vi "CRYReplace Hardware Curve Name.vi"(6 "Hardware In":string, 8 "New Name":string, 9 "Old Name":string, 10 "Type In":enum16{"Add", "Delete", "Rename"}(ring), 11 "Is Input?":bool) -> ()   [LabVIEW 2013]
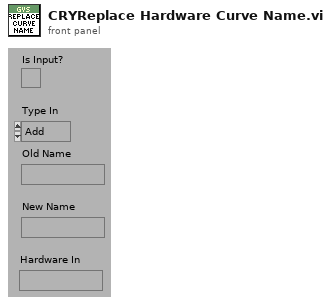
[diagram p1: front panel]
types:
  T1 = typedef "CRYStep.ctl" = cluster{"No.VI":i32, "Category":string, "StepName":string, "Seq setup flattened":string, "Comment":string, "Steps config.":bool[], "Jump config":i32[], "Start":dbl, "Increment":dbl, "Name":string, "Unit":string, "Y data":u16, "Y prefix":string, "Y dB ref":dbl, "Y unit":string, "Repeat State Array":cluster{"Start":dbl, "Increment":dbl, "Count":i32, "Num":i32}[]}
  T2 = typedef "CRYStimulus Cluster.ctl" = cluster{"StimulusType":string, "UseMLValArray":u16[], "ML_axisArray":u16[], "MLValLevelNameArray":string[], "Level(U)Array":dbl[], "Start(Stop)FreqArray":dbl[], "Start(Stop)AmpArray":dbl[], "StepResolutionArray":u16[], "Unit_Array":u16[], "DegValArray":dbl[], "DegUnitArray":string[], "Steps1":i32, "Cycle/step1(#)":u32, "Time/step1(s)":dbl, "Transition1":dbl, "SweepRate2":dbl, "Freq3(Hz)":dbl, "Steps3(#)":dbl, "Cycles3(#)":u32, "StepSize3":dbl, "wave time":string, "RMS_Value4":dbl, "Peak_Value4":dbl, "WavePath4":string, "RMS_unit4":string, "Peak_unit4":string, "wave Info":string, "dc_ctrl5_1":u16, "dc_ctrl5_2":u16, "dc_polar5":u16, "Max.Current":u16, "Steps5(#)":u32, "Time/Step5":dbl, "Level5":dbl, "StepsSize5Val":dbl, "StepSize5Unit":string, "SweepType":u16, "Fixed/Ratio6":u16, "Transition6":dbl, "Steps6(#)":dbl, "Cycle/Steps6(#)":u32, "Time/Steps6(s)":dbl, "Freq6(Hz)":dbl, "Difference6(Hz)":dbl, "Ratio6":string, "NoiseType7":u16, "Duration7(s)":dbl, "MinFreq7(Hz)":dbl, "MaxFreq7(Hz)":dbl, "MinFreq8(Hz)":dbl, "MaxFreq8(Hz)":dbl, "FreqRounding8":bool, "Duration8(s)":dbl, "Tones8":dbl, "RoundingVal8":dbl, "ApplyEQ":bool, "Duration(s)":dbl, "CustomStimulusName ":string, "Flatten Element Array":string[], "sine waves":cluster{"freq":dbl, "ampl":dbl, "cycles":dbl}[], "Channel Out":i32, "RatioVal6":dbl, "TabCtrl6":enum32{"Master Tone", "Slave Tone"}, "Signal Type Name":string, "Help":string, "Channel Sel":u16}
  T3 = typedef "CRYAcquisition Cluster.ctl" = cluster{"Mode":u16, "Name":string, "use ch name":bool, "Record Time":dbl, "hide rec":bool, "hide play":bool, "rec delay":dbl, "rec pad":dbl, "dcc units":i8, "sine gen setting":string, "scope_fft setting":string, "voltmeter setting":string, "rta setting":string, "trig offset(sec)":dbl, "triggered  record":bool, "trig level":dbl, "trig unit":u8, "trig slop":bool, "trig timeout(sec)":dbl, "add record":bool, "EQ":bool, "record table":string[][], "play table":string[][], "trig channel":string, "Help":string}
  T4 = typedef "CRYAnalysis Cluster.ctl" = cluster{"Name":string, "Harmonics":dbl[], " Algorithm":u16, "delay":dbl, "THD(%)":bool, "Rub&Buzz":bool, "Imp":bool, "Imp Ref resistor":dbl, "Y data":u16, "Y prefix":string, "Y unit":string, "Y dB ref":dbl, "Custom Curve Names":string[], "har list items":string[], "Envelope":bool, "use custom unit":bool, "autodelay ch":dbl, "impulse":bool, " start ms":dbl, " stop ms":dbl, "Scaling":i32, "Default Overlap ":bool, "Advanced View":bool, "Loose Particle":bool, "Use default":bool, "Auto-Correlation(Stimulus)":bool, "Auto-Correlation(Response)":bool, "Deconvolved Response":bool, "Mic Current":bool, "M List Vaiues":u16, "Type":u16, "Delay Method":u16, "Apply Correction Out":bool, "Apply Correction In":bool, "Harmonics @ meas.frq":bool, "THD Normalized(%)":bool, "Total Distortion":bool, "THD+Noise(%)":bool, "Rub&Buzz Norm'd(%)":bool, "Standard Error":bool, "Confidence Limits":bool, "Total Diff":bool, "Total Noise":bool, "Total DFD(%)":bool, "Total IMD(%)":bool, "Total IM":bool, "Total DFD+Noise(%)":bool, "Use Channel Name":bool, "Waveform In":string, "Waveform Out":string, "Method":u16, "Spectral Scaling":u16, "Appliied Unit":u16, "Length Unit":u16, "Applied Units":u16, "Sens Item":u16, "Tab":i32, "Distance Unit":u16, "discard cycles":dbl, "Weigting":string, "Averaging Time":dbl, "Max duration":dbl, "Min duration":dbl, "Attack Threshold":dbl, "Hysteresis Up":dbl, "Fmin(Hz)":dbl, "Fmax(Hz)":dbl, "Freq.Resolution":dbl, "Over-samples Res.":dbl, "Win Resolution":dbl, "distance":dbl, "samples":dbl, "Overlap":dbl, "Record Length":dbl, "No.of FFTs":dbl, "Hz":dbl, "record delay":dbl, " Std Err":dbl, "Response":bool, "Coherent Power*":bool, "Stimulus":bool, "Measurement Confidence":bool, "Auto Spectrum(Response)*":bool, "Auto Spectrum(Stimulus)*":bool, "Cross Spectrum*":bool, "functions":bool, "Frequency Response":bool, "Non-Coherent Power*":bool, "Coherence (%)":bool, "Non-Coherence (%)":bool, "Signal-Noise Ratio (dB)":bool, "Non-Coherenct Distirtion*":bool, "Result Waveforms":bool, "Coupling":bool, "Averaging":u16, "Harmonics":i32, "Custom Curve Names":i32, "unLabel":string, "Custom Curve Names":string, "Unit":string, "Total IMD + Noise(%) ":bool, "ResponseMe":u16, "Intermod":dbl[], "Diff\n":dbl[], "Cross-Correlation":bool, "IM list items":string[], "Diff list items":string[], "TSR Window Type":string, "Help":string, "Custom Curve IDs":i32[], "Default Curve Names":string[], "Loose Particle waveform":bool, "Perceptual Rub&Buzz":bool, "Imp Auto Mode":u16, "Mic Auto Mode":u16, "Mic Ref resistor":dbl, "Curve Resolution":u16, "Curve Resolution Hz":dbl, "Polarity":bool}
  T5 = typedef "CRYWaveform Cluster.ctl" = cluster{"Waveform":cluster{"X0":dbl, "dX":dbl, "Y":sgl[]}, "X data":u16, "Y data":u16, "Y axis":u16, "X unit":string, "Y unit":string, "Y dB ref":dbl, "display Y":bool, "display X":bool, "Overload?":bool, "Test Info":string, "Step No.":i32, "Name":string, "protected":bool, "Sqc history":string[], "Signal Channel ID":i32, "Plot Settings":cluster{"Color":u32, "Interpolation":u8, "Point Style":u8, "Line Style":u8, "Point Color":u32, "Line Width":u8, "Bar Plot Style":u8, "Fill To":i16}, "AutoProtect":bool}
  T6 = typedef "CRYStimulus Test Infor Cluster.ctl" = cluster{"Stimulus Type":string, "Signal Type":string, "In/Out":bool, "FAPS":cluster{"freq":dbl, "ampl":dbl, "cycles":dbl, "samples":i32}[], "Sampling Rate":dbl, "Samples":i32, "Analysis Param":string, "Resolution":u16, "Steps":u32, "Analysis Value":dbl[], "Diff Freq":dbl, "FStart":dbl, "FStop":dbl, "Calibration Param":string, "Anti Alias":dbl, "Level Out1":dbl, "Level Out2":dbl, "EQ":bool}
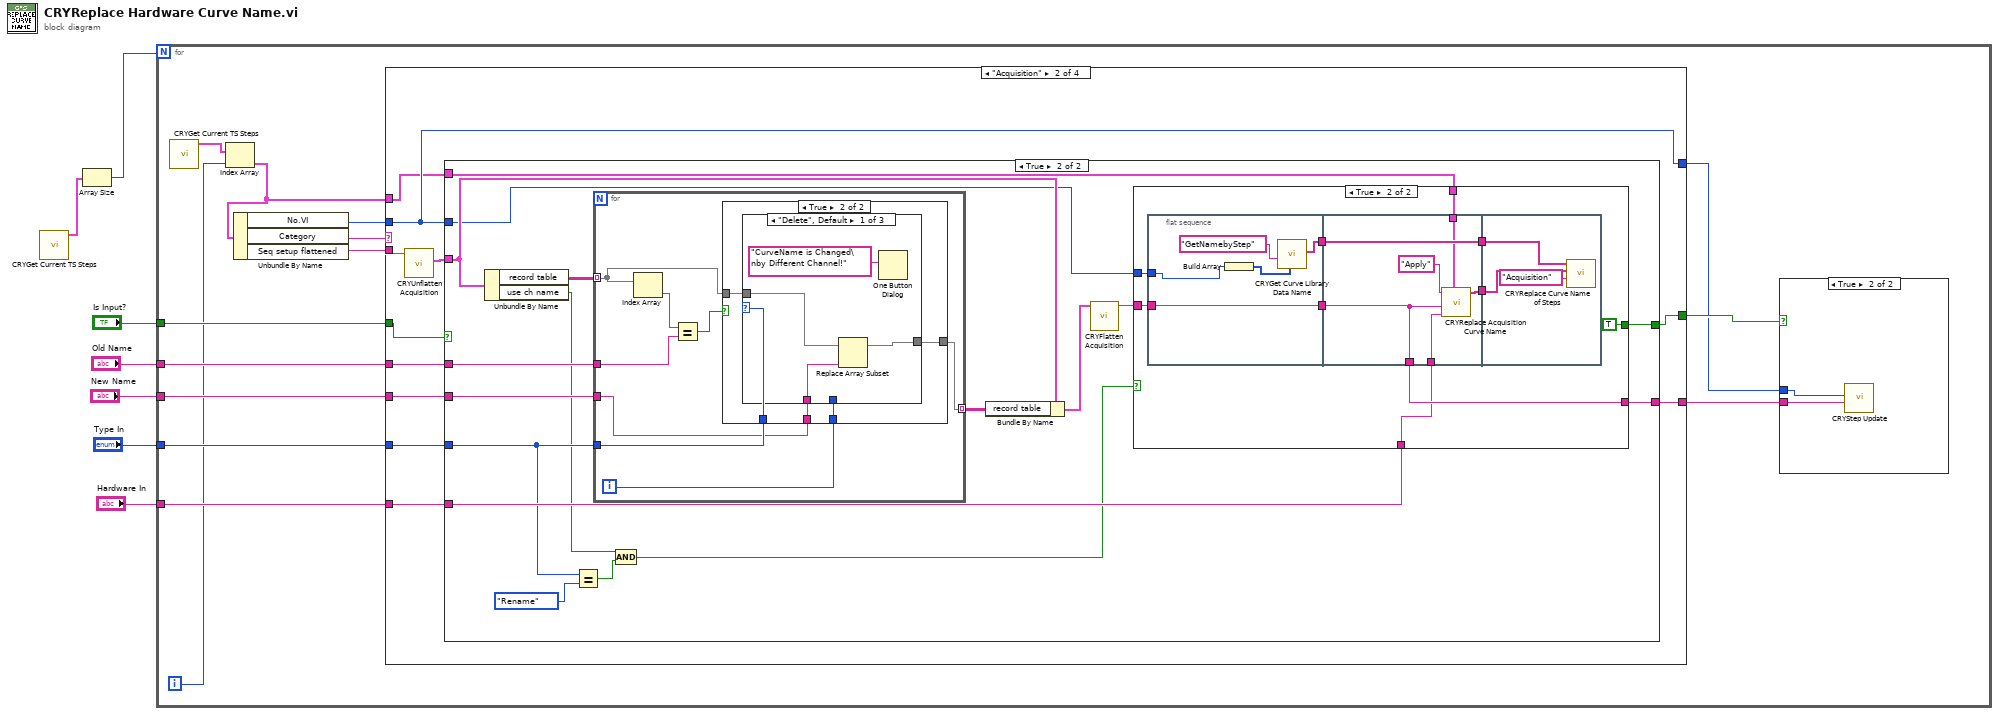
[diagram p0: block diagram]
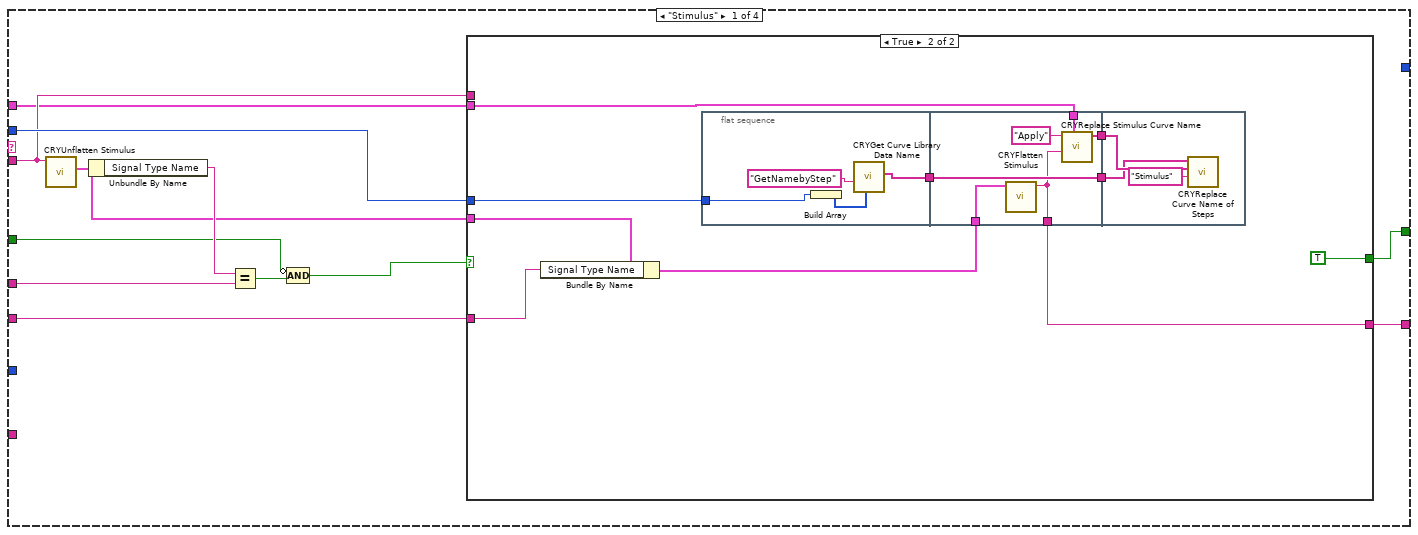
[diagram p3: hidden frame]
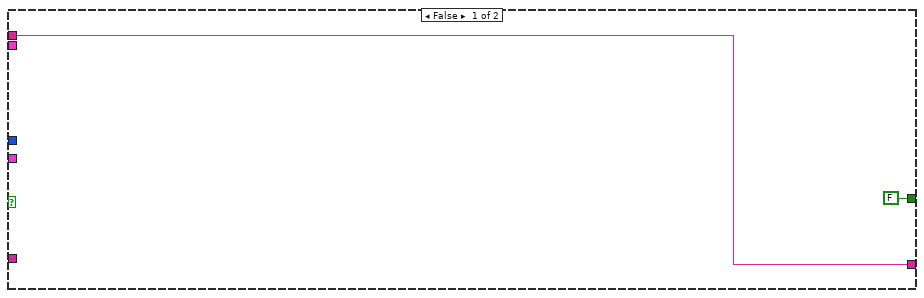
[diagram p4: hidden frame]
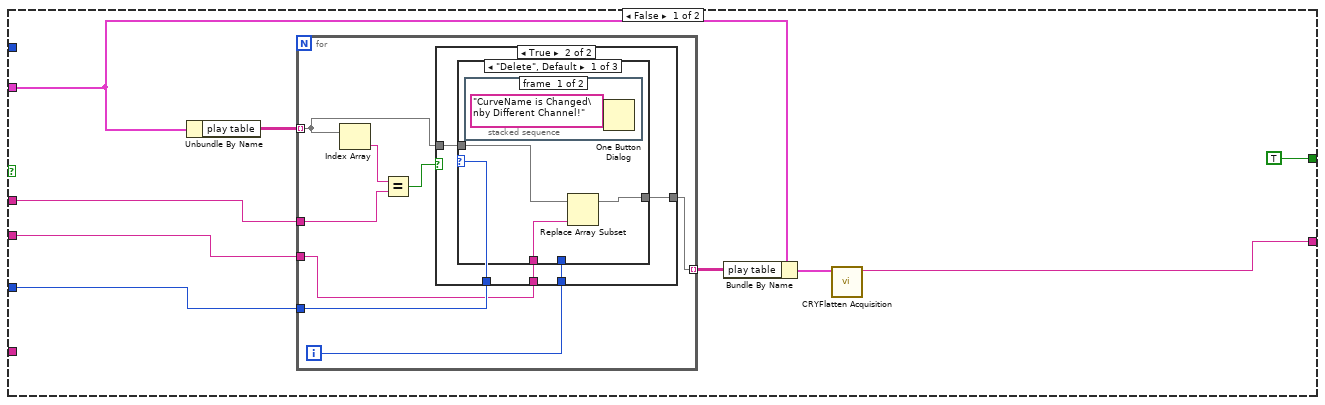
[diagram p5: hidden frame]
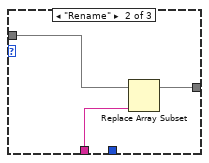
[diagram p8: hidden frame]
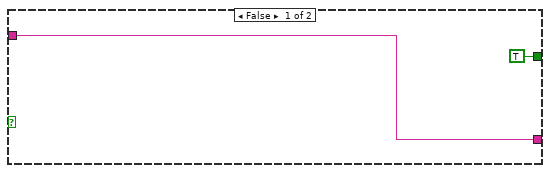
[diagram p10: hidden frame]
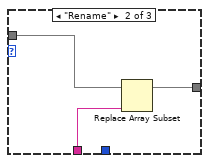
[diagram p12: hidden frame]
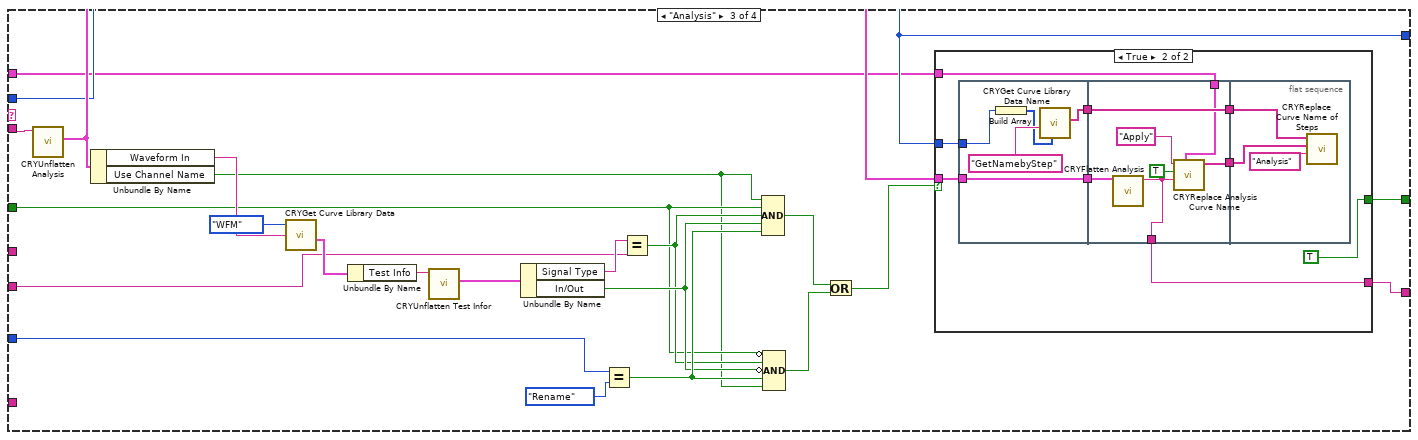
[diagram p14: hidden frame]
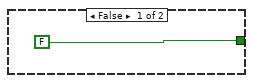
[diagram p15: hidden frame]
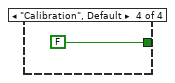
[diagram p16: hidden frame]
diagram:
  n1 = call "CRYGet Current TS Steps.vi"() -> ("Steps"=w2:T1[])  [unwired: 7 in, 4 out]
  n2 = Array Size(array=w2) -> (size(s)=w1:i32)
  n3 = for {
    N: w1 -> [_]
    tunnel: "Is Input?" -> [w19]
    tunnel: "Old Name" -> [w18]
    tunnel: "Type In" -> [w17]
    tunnel: "New Name" -> [w16]
    tunnel: "Hardware In" -> [w14]
    i -> [w9]
    n4 = call "CRYGet Current TS Steps.vi"() -> ("Steps"=w10:T1[])  [unwired: 7 in, 4 out]
    n5 = Index Array(array=w10, index=w9) -> (element=w8:T1)
    n6 = Unbundle By Name(w8) -> ("No.VI"=w13:i32, "Category"=w21:string, "Seq setup flattened"=w20:string)
    n7 = case shown="\"Acquisition\"" w21 {
      tunnel: w20 -> [w26 w66 w188 _]
      tunnel: w19 -> [w31 w71 w174 _]
      tunnel: w18 -> [w33 w70 _ _]
      tunnel: w17 -> [_ w69 w179 _]
      tunnel: w16 -> [w28 w68 w169 _]
      tunnel: [w27 w65 w190 _] -> w15
      tunnel: w14 -> [_ w64 _ _]
      tunnel: w13 -> [w35 w62 w180 _]
      tunnel: [w25 w63 w189 FALSE] -> w12
      tunnel: [_ w62 w180 _] -> w11
      tunnel: w8 -> [w24 w61 w168 _]
      frame "Stimulus" {
        n8 = call "CRYUnflatten Stimulus.vi"("Flatten Stimulus"=w26) -> ("Stimulus"=w29:T2)  [unwired: 8 in, 2 out]
        n9 = Unbundle By Name(w29) -> ("Signal Type Name"=w34:string)
        n10 = Equal?(x=w34, y=w33) -> (x = y?=w32:bool)
        n11 = Compound Arithmetic op=AND(invert w31, w32) -> (w30:bool)
        n12 = case shown="True" w30 {
          tunnel: w35 -> [_ w44]
          tunnel: w29 -> [_ w43]
          tunnel: w28 -> [_ w42]
          tunnel: [w37 w40] -> w27
          tunnel: w26 -> [w37 _]
          tunnel: [FALSE TRUE] -> w25
          tunnel: w24 -> [_ w38]
          frame False {
          }
          frame True {
            n13 = Bundle By Name(cluster=w43, "Signal Type Name"=w42) -> (w41:T2)
            n14 = flat-sequence {
              tunnel: [w50] -> w47
              tunnel: w44 -> [w49]
              tunnel: [w56] -> w46
              tunnel: [w55] -> w45
              tunnel: w47 -> [w55]
              tunnel: w41 -> [w54]
              tunnel: [w53] -> w40
              tunnel: w38 -> [w52]
              tunnel: w46 -> [w59]
              tunnel: w45 -> [w58]
              frame #0 {
                n15 = Build Array(w49) -> (w48:i32[])
                n16 = call "CRYGet Curve Library Data Name.vi"("nData"=w48, "sOption"="GetNamebyStep") -> ("sNames"=w50:string[])  [unwired: 6 in, 3 out]
              }
              frame #1 {
                n17 = call "CRYFlatten Stimulus.vi"("Stimulus"=w54) -> ("Flatten Stimulus String"=w53:string)  [unwired: 10 in]
                n18 = call "CRYReplace Stimulus Curve Name.vi"("Setup in"=w52, "Step Setup In"=w53, "Type In"="Apply" ("Type")) -> ("Inserted Names Out"=w56:string[])  [unwired: 8 in]
              }
              frame #2 {
                n19 = call "CRYReplace Curve Name of Steps.vi"("Step Category"="Stimulus", "New Name"=w59, "Old Name"=w58) -> ()  [unwired: 8 in, 1 out]
              }
            }
          }
        }
      }
      frame "Acquisition" {
        n20 = call "CRYUnflatten Acquisition.vi"("Flatten Acquisition"=w66) -> ("Acquisition"=w67:T3)  [unwired: 10 out]
        n21 = case shown="True" w71 {
          tunnel: w70 -> [w78 w118]
          tunnel: w69 -> [w76 w109]
          tunnel: w68 -> [w77 w117]
          tunnel: w67 -> [w75 w115]
          tunnel: [w72 w114] -> w65
          tunnel: w64 -> [_ w112]
          tunnel: w62 -> [_ w113]
          tunnel: [TRUE w111] -> w63
          tunnel: w61 -> [_ w103]
          frame False {
            n22 = Unbundle By Name(w75) -> ("play table"=w79:string[][])
            n23 = for {
              tunnel: w79 -> [w84] mode=indexing
              tunnel: w78 -> [w88]
              tunnel: w76 -> [w86]
              tunnel: w77 -> [w83]
              tunnel: [w81] -> w74 mode=indexing
              i -> [w82]
              n24 = Index Array(array=w84) -> (element=w85:string)  [unwired: 1 in]
              n25 = Equal?(x=w85, y=w88) -> (x = y?=w87:bool)
              n26 = case shown="True" w87 {
                tunnel: w86 -> [_ w94]
                tunnel: w84 -> [w89 w93]
                tunnel: w83 -> [_ w92]
                tunnel: [w89 w91] -> w81
                tunnel: w82 -> [_ w90]
                frame False {
                }
                frame True {
                  n27 = case shown="\"Delete\", Default" w94 {
                    tunnel: w93 -> [w97 w101 w102]
                    tunnel: w92 -> [w96 w100 _]
                    tunnel: [w95 w99 w102] -> w91
                    tunnel: w90 -> [_ _ _]
                    frame "Delete", Default {
                      n28 = stacked-sequence {
                        frame #0 {
                          n29 = One Button Dialog(message="CurveName is Changed\nby Different Channel!") -> ()  [unwired: 2 out]
                        }
                        frame #1 {
                        }
                      }
                      n30 = Replace Array Subset(array=w97, new element=w96) -> (w95:string[])  [unwired: 1 in]
                    }
                    frame "Rename" {
                      n31 = Replace Array Subset(array=w101, new element=w100) -> (w99:string[])  [unwired: 1 in]
                    }
                    frame "Add" {
                    }
                  }
                }
              }
            }
            n32 = Bundle By Name(cluster=w75, "play table"=w74) -> (w73:T3)
            n33 = call "CRYFlatten Acquisition.vi"("Acquisition"=w73) -> ("Acquisition flattened"=w72:string)  [unwired: 10 out]
          }
          frame True {
            n34 = Unbundle By Name(w115) -> ("record table"=w119:string[][], "use ch name"=w108:bool)
            n35 = Equal?(x=w109, y=enum16{"Add", "Delete", "Rename"}."Rename" ("Type In")) -> (x = y?=w107:bool)
            n36 = for {
              tunnel: w119 -> [w149] mode=indexing
              tunnel: w118 -> [w153]
              tunnel: w109 -> [w151]
              tunnel: w117 -> [w148]
              tunnel: [w146] -> w116 mode=indexing
              i -> [w147]
              n37 = Index Array(array=w149) -> (element=w150:string)  [unwired: 1 in]
              n38 = Equal?(x=w150, y=w153) -> (x = y?=w152:bool)
              n39 = case shown="True" w152 {
                tunnel: w151 -> [_ w159]
                tunnel: w149 -> [w154 w158]
                tunnel: w148 -> [_ w157]
                tunnel: [w154 w156] -> w146
                tunnel: w147 -> [_ w155]
                frame False {
                }
                frame True {
                  n40 = case shown="\"Delete\", Default" w159 {
                    tunnel: w158 -> [w163 w166 w167]
                    tunnel: w157 -> [w162 w165 _]
                    tunnel: [w161 w164 w167] -> w156
                    tunnel: w155 -> [_ _ _]
                    frame "Delete", Default {
                      n41 = Replace Array Subset(array=w163, new element=w162) -> (w161:string[])  [unwired: 1 in]
                      n42 = One Button Dialog(message="CurveName is Changed\nby Different Channel!") -> ()  [unwired: 2 out]
                    }
                    frame "Rename" {
                      n43 = Replace Array Subset(array=w166, new element=w165) -> (w164:string[])  [unwired: 1 in]
                    }
                    frame "Add" {
                    }
                  }
                }
              }
            }
            n44 = Compound Arithmetic op=AND(w108, w107) -> (w106:bool)
            n45 = Bundle By Name(cluster=w115, "record table"=w116) -> (w105:T3)
            n46 = call "CRYFlatten Acquisition.vi"("Acquisition"=w105) -> ("Acquisition flattened"=w104:string)  [unwired: 10 out]
            n47 = case shown="True" w106 {
              tunnel: w104 -> [w120 w127]
              tunnel: [w120 w126] -> w114
              tunnel: w113 -> [_ w125]
              tunnel: w112 -> [_ w124]
              tunnel: [TRUE TRUE] -> w111
              tunnel: w103 -> [_ w122]
              frame False {
              }
              frame True {
                n48 = flat-sequence {
                  tunnel: w127 -> [w136]
                  tunnel: [w134] -> w131
                  tunnel: [w136] -> w130
                  tunnel: w125 -> [w133]
                  tunnel: [w142] -> w129
                  tunnel: w124 -> [w139]
                  tunnel: [w141] -> w128
                  tunnel: w131 -> [w142]
                  tunnel: w130 -> [w138]
                  tunnel: [w138] -> w126
                  tunnel: w122 -> [w137]
                  tunnel: w129 -> [w144]
                  tunnel: w128 -> [w143]
                  frame #0 {
                    n49 = Build Array(w133) -> (w132:i32[])
                    n50 = call "CRYGet Curve Library Data Name.vi"("nData"=w132, "sOption"="GetNamebyStep") -> ("sNames"=w134:string[])  [unwired: 6 in, 3 out]
                  }
                  frame #1 {
                    n51 = call "CRYReplace Acquisition Curve Name.vi"("Setup in"=w137, "Hardware Setup In"=w139, "Step Setup In"=w138, "Type In"="Apply") -> ("Inserted Names Out"=w141:string[])  [unwired: 5 in, 2 out]
                  }
                  frame #2 {
                    n52 = call "CRYReplace Curve Name of Steps.vi"("Step Category"="Acquisition", "New Name"=w143, "Old Name"=w144) -> ()  [unwired: 8 in, 1 out]
                  }
                }
              }
            }
          }
        }
      }
      frame "Analysis" {
        n53 = call "CRYUnflatten Analysis.vi"("Unflatten Analysis"=w188) -> ("Analysis"=w181:T4)  [unwired: 8 in, 2 out]
        n54 = Unbundle By Name(w181) -> ("Waveform In"=w187:string, "Use Channel Name"=w170:bool)
        n55 = call "CRYGet Curve Library Data.vi"("Type"=enum16{"Curves", "Values", "Results", "WFM"}."WFM", "Data Name"=w187) -> ("Wave"=w185:T5)  [unwired: 4 out]
        n56 = Unbundle By Name(w185) -> ("Test Info"=w184:string)
        n57 = call "CRYUnflatten Test Infor.vi"("Falattend test infor"=w184) -> ("unflattened test infor data"=w183:T6)  [unwired: 9 out]
        n58 = Unbundle By Name(w183) -> ("Signal Type"=w182:string, "In/Out"=w176:bool)
        n59 = Equal?(x=w179, y=enum16{"Add", "Delete", "Rename"}."Rename" ("Type In")) -> (x = y?=w177:bool)
        n60 = Equal?(x=w182, y=w169) -> (x = y?=w175:bool)
        n61 = Compound Arithmetic op=AND(w170, w174, w175, w176, w177) -> (w173:bool)
        n62 = Compound Arithmetic op=AND(invert w174, w175, invert w176, w177, w170) -> (w172:bool)
        n63 = Or(x=w173, y=w172) -> (x .or. y?=w171:bool)
        n64 = case shown="True" w171 {
          tunnel: w181 -> [_ w196]
          tunnel: [_ w195] -> w190
          tunnel: w180 -> [_ w194]
          tunnel: [FALSE TRUE] -> w189
          tunnel: w168 -> [_ w192]
          frame False {
          }
          frame True {
            n65 = flat-sequence {
              tunnel: w196 -> [w205]
              tunnel: [w201] -> w200
              tunnel: [w205] -> w199
              tunnel: w194 -> [w203]
              tunnel: [w212] -> w198
              tunnel: [w211] -> w197
              tunnel: w200 -> [w212]
              tunnel: w199 -> [w208]
              tunnel: [w210] -> w195
              tunnel: w192 -> [w207]
              tunnel: w198 -> [w214]
              tunnel: w197 -> [w213]
              frame #0 {
                n66 = Build Array(w203) -> (w202:i32[])
                n67 = call "CRYGet Curve Library Data Name.vi"("nData"=w202, "sOption"="GetNamebyStep") -> ("sNames"=w201:string[])  [unwired: 6 in, 3 out]
              }
              frame #1 {
                n68 = call "CRYFlatten Analysis.vi"("Analysis"=w208) -> ("Analysis flattened"=w210:string)  [unwired: 10 in]
                n69 = call "CRYReplace Analysis Curve Name.vi"("Setup in"=w207, "Step Setup In"=w210, "InsertSocket?"=TRUE, "Type In"="Apply") -> ("Inserted Names Out"=w211:string[])  [unwired: 3 in, 4 out]
              }
              frame #2 {
                n70 = call "CRYReplace Curve Name of Steps.vi"("Step Category"="Analysis", "New Name"=w213, "Old Name"=w214) -> ()  [unwired: 8 in, 1 out]
              }
            }
          }
        }
      }
      frame "Calibration", Default {
      }
    }
    n71 = case shown="True" w12 {
      tunnel: w15 -> [_ w23]
      tunnel: w11 -> [_ w22]
      frame False {
      }
      frame True {
        n72 = call "CRYStep Update.vi"("Seq-step setup"=w23, "Proper VI No"=w22) -> ()  [unwired: 10 in]
      }
    }
  }
